vi "Cannon Modifications.vi"(1 "Cannon Global Data In":T2) -> (0 "Cannon Global Data Out":T2)   [LabVIEW 2013]
uses:
  <vilib>/Rock Robotics/WPI/Solenoid/WPI_SolenoidValue.ctl
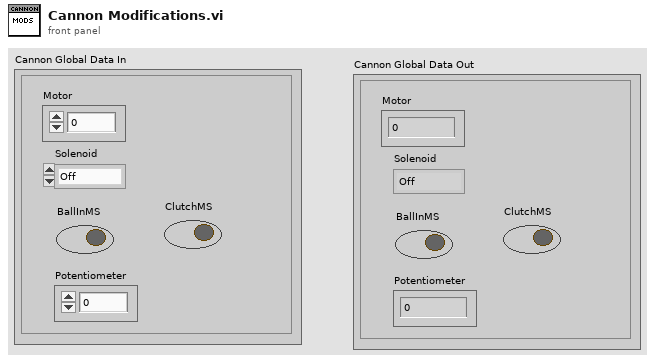
[diagram p1: front panel]
types:
  T1 = typedef "WPI_SolenoidValue.ctl" = enum16{"Off", "On", "Forward", "Reverse"}
  T2 = cluster{"Motor":dbl, "Solenoid":T1, "BallInMS":bool, "ClutchMS":bool, "Potentiometer":dbl}
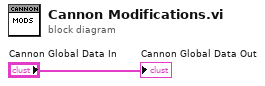
[diagram p0: block diagram]
diagram:
  "Cannon Global Data Out" <- "Cannon Global Data In"
